vi "Utility Read From Register - Floating Point.vi"(0 "VISA resource name":refnum<visa-resource-name>, 1 "Unit Address (1)":u8=1, 5 "Register Address (0)":u16, 9 "Num Of Reg (1)":u16=1 min=1 step=1, 11 "error in (no error)":errorcluster) -> (4 "VISA resource name out":refnum<visa-resource-name>, 6 "Data":sgl[](array[numeric]) format="%.3f", 15 "error out":errorcluster)   [LabVIEW 2010, in "Eurotherm 32xx Series.lvlib"]
doc: "This VI reads value from specified registers of specified unit."
uses:
  <instrlib>/Eurotherm 32xx Series/Eurotherm 32xx Series.lvlib
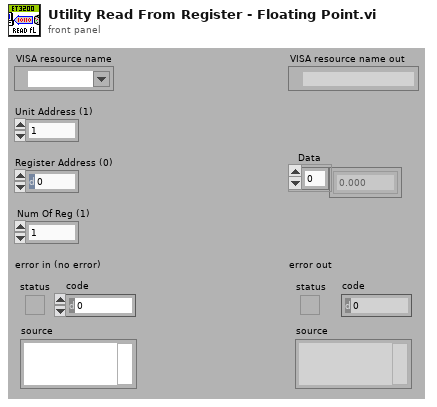
[diagram p1: front panel]
types:
  T1 = enum16{"By The Number of Bytes", "Copy Of the Sent Message"}
  T2 = cluster{"Read Buffer[0]":u8, "Read Buffer[1]":u8}
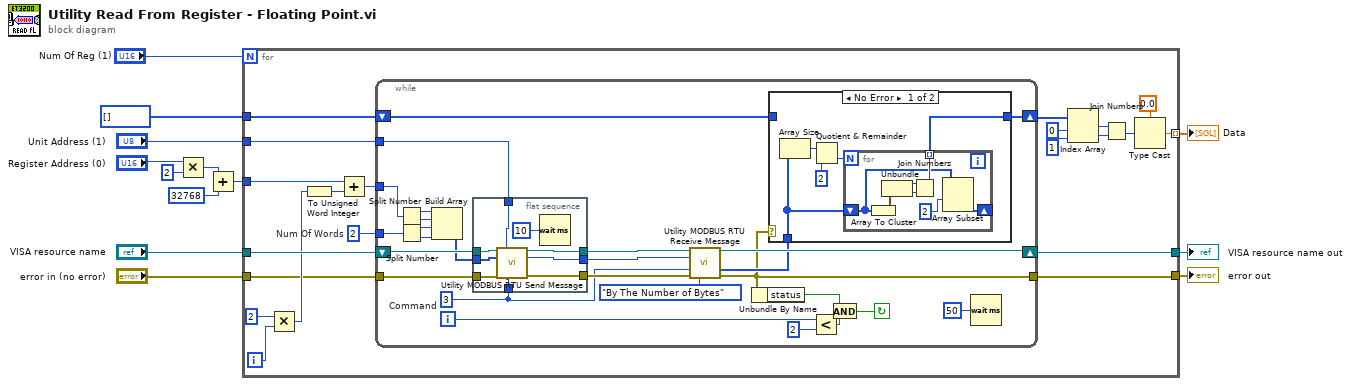
[diagram p0: block diagram]
diagram:
  n1 = Multiply(x="Register Address (0)", y=u16 2) -> (x*y=w6:u16)
  n2 = Add(x=w6, y=u16 32768) -> (x+y=w1:u16)
  n3 = for {
    N: "Num Of Reg (1)" -> [_]
    tunnel: "VISA resource name" -> [w34]
    tunnel: [w33] -> w12
    tunnel: u16[] [] -> [w32]
    tunnel: "error in (no error)" -> [w15]
    tunnel: [w14] -> w9
    tunnel: "Unit Address (1)" -> [w31]
    tunnel: w1 -> [w21]
    tunnel: [w23] -> w2 mode=indexing
    i -> [w20]
    w30 = u16 2  # Num Of Words
    n4 = Multiply(x=2, y=w20) -> (x*y=w18:i32)
    n5 = To Unsigned Word Integer(number=w18) -> (unsigned 16bit integer=w17:u16)
    n6 = Add(x=w21, y=w17) -> (x+y=w22:u16)
    n7 = while {
      tunnel: w31 -> [w41]
      shift-right: [w57] -> w33
      shift-left: w34 -> [w58]
      tunnel: w30 -> [w44]
      shift-right: [w46] -> w16
      shift-left: w32 -> [w45]
      tunnel: w22 -> [w37]
      tunnel: w15 -> [w36]
      tunnel: [w35] -> w14
      i -> [w53]
      stop <- w55 continue-if-true
      w54 = u8 3  # Command
      n8 = Split Number(x=w37) -> (hi(x)=w49:u8, lo(x)=w48:u8)
      n9 = Split Number(x=w44) -> (hi(x)=w43:u8, lo(x)=w42:u8)
      n10 = Build Array(w49, w48, w43, w42) -> (w50:u8[])
      n11 = flat-sequence {
        tunnel: [w69] -> w60
        tunnel: [w68] -> w59
        tunnel: w58 -> [w67]
        tunnel: w54 -> [w66]
        tunnel: w50 -> [w65]
        tunnel: w41 -> [w64]
        tunnel: [w63] -> w39
        tunnel: w36 -> [w62]
        frame #0 {
          n12 = call <instrlib>:"Utility MODBUS RTU Send Message.vi"("VISA resource name"=w67, "Unit Address (1)"=w64, "Message (empty array)"=w65, "error in (no error)"=w62, "Command (0)"=w66) -> ("VISA resource name out"=w68:refnum<visa-resource-name>, "Length Of Sent MSG"=w63:u8, "error out"=w69:errorcluster)  [unwired: 8 in]
          n13 = Wait (ms)(milliseconds to wait=u32 10) -> ()  [unwired: 1 out]
        }
      }
      n14 = call <instrlib>:"Utility MODBUS RTU Receive Message.vi"("VISA resource name"=w59, "Length Of Sent MSG (0)"=w39, "Sent Command (0)"=w54, "error in (no error)"=w60, "Receive Message Type (0: By The Number Of Bytes)"=T1."By The Number of Bytes" ("Receive Message Type")) -> ("VISA resource name out"=w57:refnum<visa-resource-name>, "Read Buffer"=w47:u8[], "error out"=w35:errorcluster)  [unwired: 8 in]
      n15 = Unbundle By Name(w35) -> ("status"=w56:bool)
      n16 = case shown="No Error" w35 {
        tunnel: w47 -> [w74 _]
        tunnel: [w73 w82] -> w46
        tunnel: w45 -> [_ w82]
        frame No Error {
          n17 = Array Size(array=w74) -> (size(s)=w72:i32)
          n18 = Quotient & Remainder(x=w72, y=2) -> (floor(x/y)=w70:i32)  [unwired: 1 out]
          n19 = for {
            N: w70 -> [_]
            shift-right: [w76] -> _
            shift-left: w74 -> [w77]
            tunnel: [w78] -> w73 mode=indexing
            n20 = Array To Cluster(array=w77) -> (cluster=w81:T2)
            n21 = Unbundle(w81) -> ("Read Buffer[0]"=w79:u8, "Read Buffer[1]"=w80:u8)
            n22 = Join Numbers(hi=w79, lo=w80) -> ((hi.lo)=w78:u16)
            n23 = Array Subset(array=w77, index=2) -> (w76:u8[])  [unwired: 1 in]
          }
        }
        frame Error {
        }
      }
      n24 = Less?(x=w53, y=2) -> (x < y?=w52:bool)
      n25 = And(x=w56, y=w52) -> (x .and. y?=w55:bool)
      n26 = Wait (ms)(milliseconds to wait=u32 50) -> ()  [unwired: 1 out]
    }
    n27 = Index Array(array=w16, index #1=0 ("index"), index #2=1 ("index")) -> (element #1=w28:u16, element #2=w29:u16)
    n28 = Join Numbers(hi=w28, lo=w29) -> ((hi.lo)=w24:u32)
    n29 = Type Cast(type=sgl 0.0, x=w24) -> (*(type *) &x=w23:sgl)
  }
  "error out" <- w9
  "VISA resource name out" <- w12
  "Data" <- w2
